vi "ASI Get Num Of Connected Cameras.vi"() -> (3 "function return":i32)   [LabVIEW 2012, in "ASICamera2_no_err.lvlib"]
doc: "ASICAMERA_API int ASIGetNumOfConnectedCameras();"
uses:
  <userlib>/ASICamera2_no_err/ASICamera2_no_err.lvlib
  ASICamera2.dll
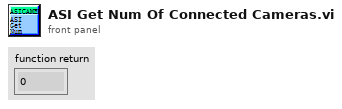
[diagram p1: front panel]
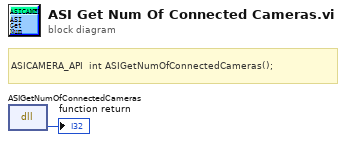
[diagram p0: block diagram]
diagram:
  # "ASICAMERA_API  int ASIGetNumOfConnectedCameras();"
  n1 = dll-call lib="ASICamera2.*" fn="ASIGetNumOfConnectedCameras"() -> (→"function return":i32)  [unwired: 3 in, 2 out]
